vi "Reverse 1D Array.vi"(8 "error in (no error)":errorcluster, 11 "JSON Value in":refnum<class "JSON Value.lvclass">) -> (0 "error out":errorcluster, 3 "JSON Value out":refnum<class "JSON Value.lvclass">)   [LabVIEW 2017, in "JSON Value.lvclass"]
doc: "Reverses the order of the elements in array, where array is of any type."
uses:
  JSON Value.lvclass
  JSON Value.lvclass/JSON Value.ctl
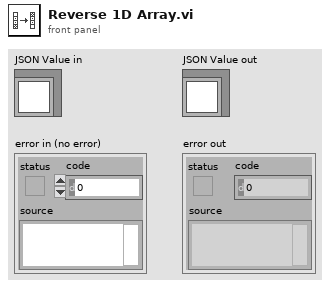
[diagram p1: front panel]
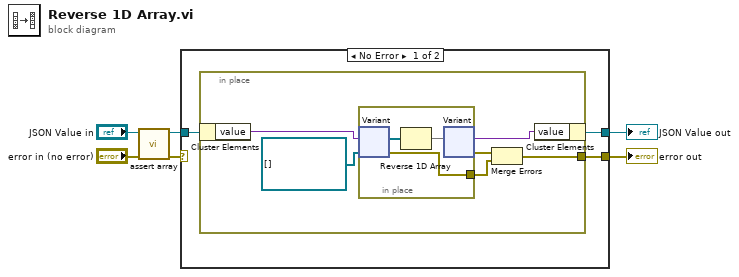
[diagram p0: block diagram]
diagram:
  n1 = call "assert array.vi"("error in (no error)"="error in (no error)", "JSON Value in"="JSON Value in") -> ("error out"=w2:errorcluster, "JSON Value out"=w4:refnum<class "JSON Value.lvclass">)  [unwired: 8 in]
  n2 = case shown="No Error" w2 {
    selector: w2 -> [_ w19]
    tunnel: [w9 w20] -> w5
    tunnel: w4 -> [w8 w20]
    tunnel: [w7 w19] -> w1
    frame No Error {
      n3 = in-place {
        in-place-border: [w10] -> w7
        n4 = in-place-cluster #1(w8) -> ("value"=w14:variant)
        n5 = in-place {
          in-place-border: [w16] -> w11
          n6 = in-place-variant #2(w14, refnum<class "JSON Value.lvclass">[] [] ("JSON Value in")) -> (w18:refnum<class "JSON Value.lvclass">[], w16:errorcluster)
          n7 = Reverse 1D Array(array=w18) -> (reversed array=w17:refnum<class "JSON Value.lvclass">[])
          n8 = in-place-variant #2(w17) -> (w13:variant, w12:errorcluster)
        }
        n9 = Merge Errors(w12, w11) -> (w10:errorcluster)
        n10 = in-place-cluster #1("value"=w13) -> (w9:refnum<class "JSON Value.lvclass">)
      }
    }
    frame Error {
    }
  }
  "JSON Value out" <- w5
  "error out" <- w1
